vi "testGetConnStatusFromServersAandB.vi"(8 "error in":errorcluster) -> (0 "error out":errorcluster)   [LabVIEW 2018]
doc: "User can not get the connStatus boolean from two TCP/IP servers because runServer.vi can not run at same time."
uses:
  <vilib>/addons/_JKI Toolkits/Caraya/classes/Assert/Assert Equal Value_Variant.vi
  src/TcpServer/TcpServer.lvclass
  <vilib>/addons/_JKI Toolkits/Caraya/classes/Test/Test.lvclass
  <vilib>/addons/_JKI Toolkits/Caraya/classes/Assert/Assert.lvclass
panel:
  out "Run Server B error out":errorcluster
  out "Run Server A error out":errorcluster
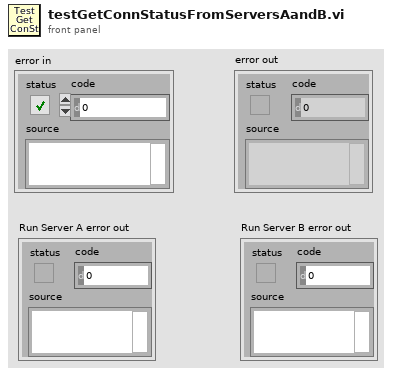
[diagram p1: front panel]
types:
  T1 = cluster{"CmdRead":refnum<user-event>, "EvtRead":refnum<user-event>, "GenRead":refnum<user-event>}
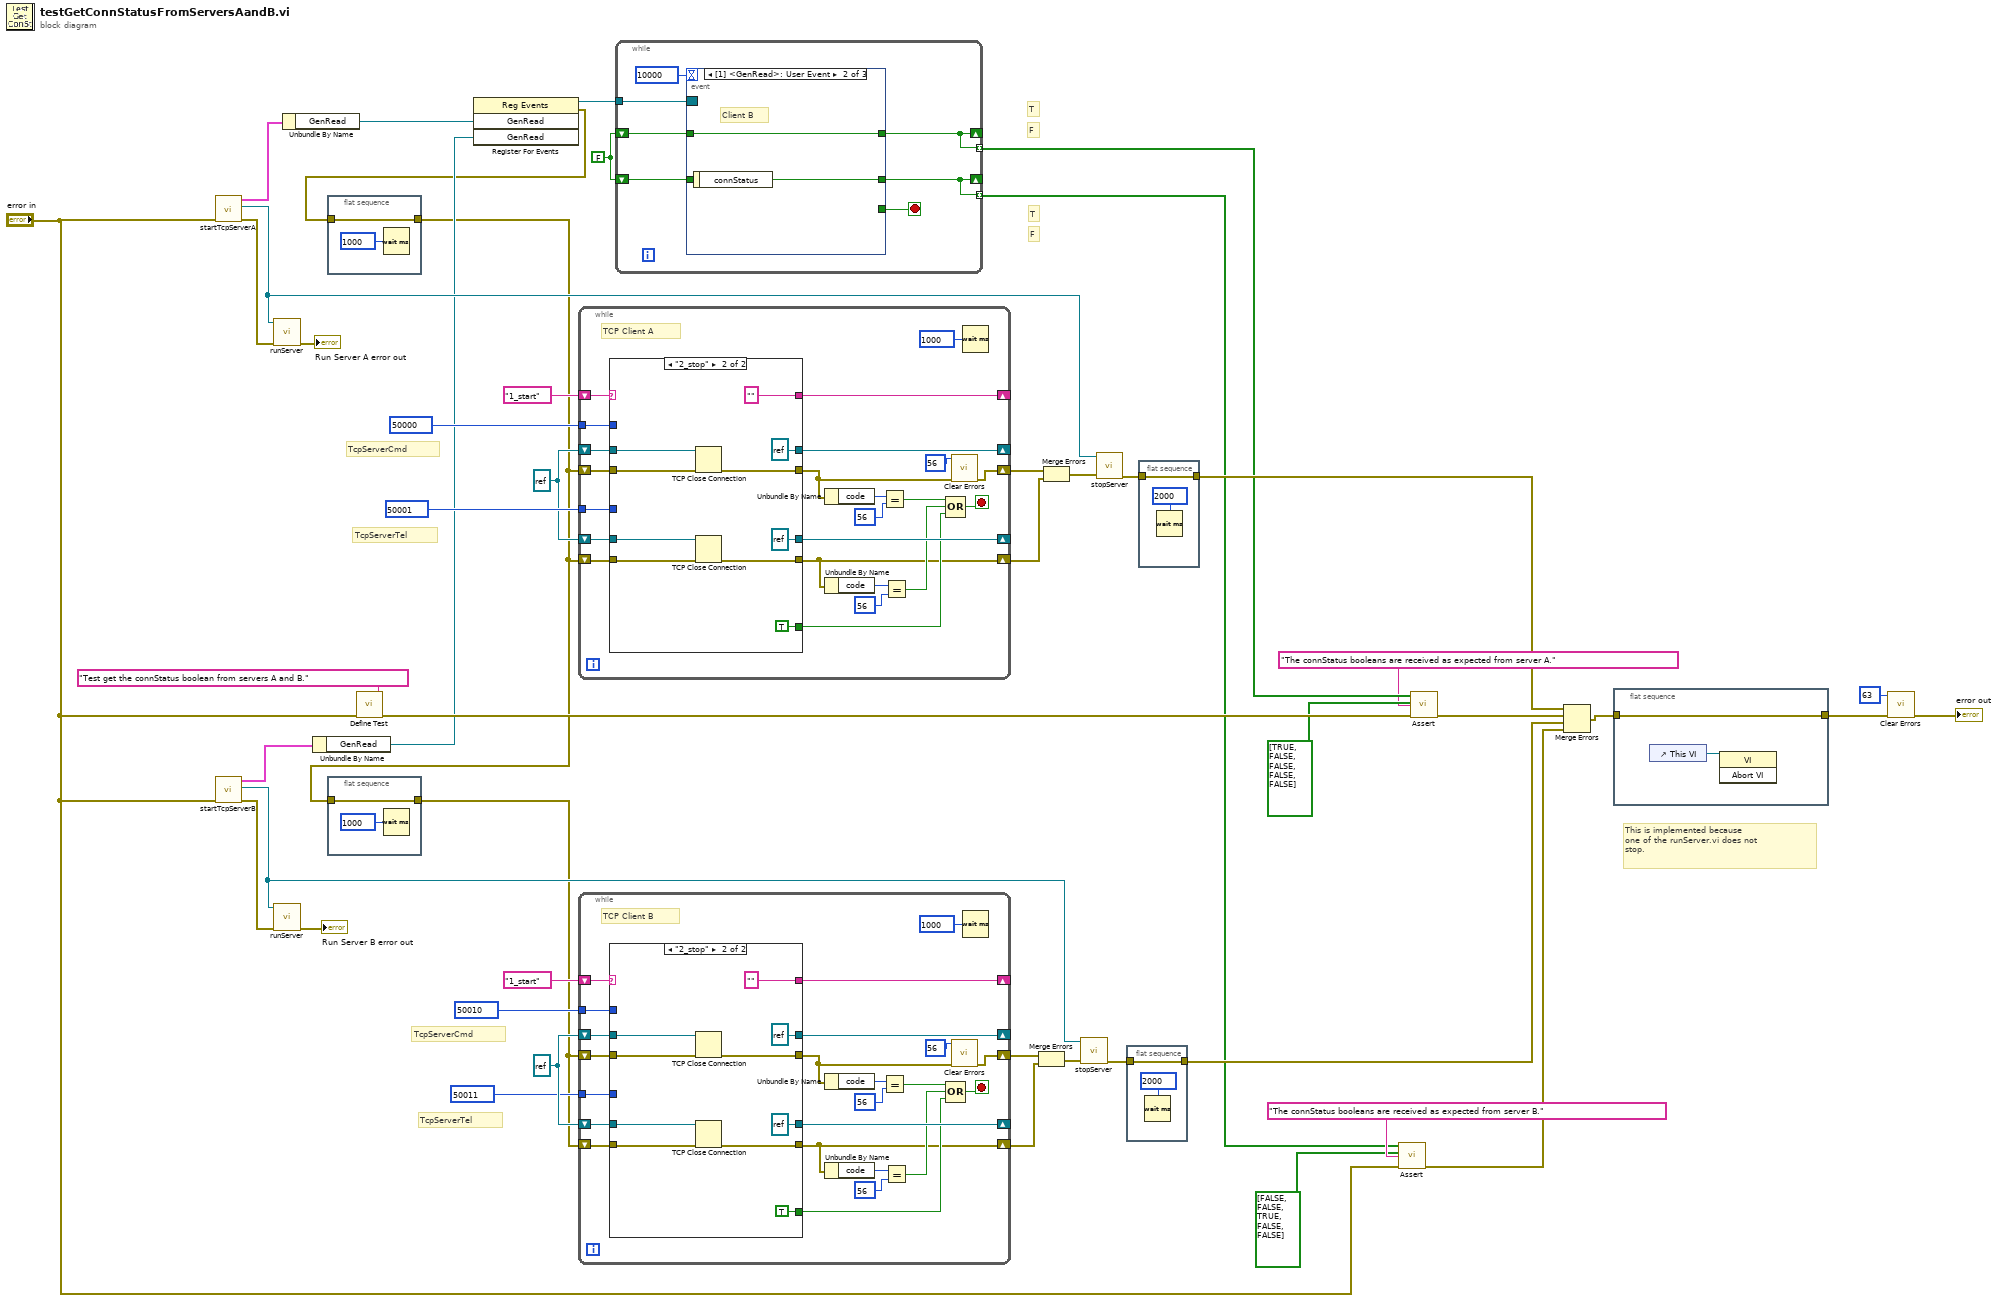
[diagram p0: block diagram]
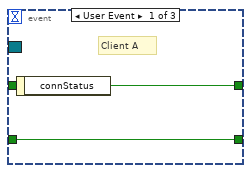
[diagram p2: hidden frame]
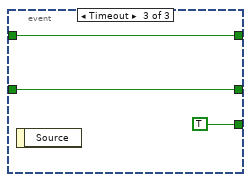
[diagram p3: hidden frame]
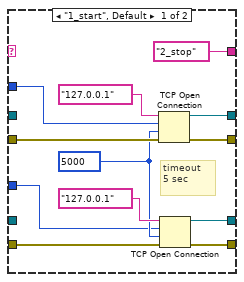
[diagram p4: hidden frame]
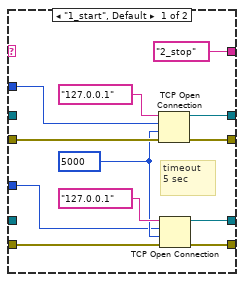
[diagram p5: hidden frame]
diagram:
  w18 = FALSE ("connStatus")
  w35 = refnum<k5> refnum ("connection ID")
  w37 = refnum<k5> refnum ("connection ID")
  # "F"
  # "F"
  # "T"
  # "T"
  # "This is implemented because\none of the runServer.vi does not\nstop."
  # "TcpServerTel"
  # "TcpServerCmd"
  # "TcpServerTel"
  # "TcpServerCmd"
  n1 = call "startTcpServerA.vi"("error in (no error)"="error in") -> ("error out"=w38:errorcluster, "TcpServer out"=w36:refnum<class "TcpServer.lvclass">, "UserEvents"=w24:T1)  [unwired: 8 in]
  n2 = call "startTcpServerB.vi"("error in (no error)"="error in") -> ("error out"=w26:errorcluster, "TcpServer out"=w28:refnum<class "TcpServer.lvclass">, "UserEvents"=w20:T1)  [unwired: 8 in]
  n3 = call "runServer.vi"("error in (no error)"=w38, "TcpServer in"=w36) -> ("error out (no error)"=→"Run Server A error out":errorcluster)  [unwired: 8 in, 1 out]
  n4 = call "runServer.vi"("error in (no error)"=w26, "TcpServer in"=w28) -> ("error out (no error)"=→"Run Server B error out":errorcluster)  [unwired: 8 in, 1 out]
  n5 = Unbundle By Name(w24) -> ("GenRead"=w23:refnum<user-event>)
  n6 = Unbundle By Name(w20) -> ("GenRead"=w19:refnum<user-event>)
  n7 = flat-sequence {
    tunnel: w7 -> [w49]
    tunnel: [w49] -> w6
    frame #0 {
      n8 = Wait (ms)(milliseconds to wait=u32 1000) -> ()  [unwired: 1 out]
    }
  }
  n9 = flat-sequence {
    tunnel: w6 -> [w51]
    tunnel: [w51] -> w27
    frame #0 {
      n10 = Wait (ms)(milliseconds to wait=u32 1000) -> ()  [unwired: 1 out]
    }
  }
  n11 = call <vilib>:"Define Test.vi"("error in (no error)"="error in", "Label (VI Title)"="Test get the connStatus boolean from servers A and B.") -> ("error out"=w40:errorcluster)  [unwired: 9 in]
  n12 = register-events(w23, w19) -> (reference out=w22:refnum<event-registration>, error out=w7:errorcluster)  [unwired: 2 in]
  n13 = while {
    shift-right: [w68] -> _
    shift-left: "1_start" ("address") -> [w75]
    shift-right: [w74] -> _
    shift-left: w37 -> [w72]
    shift-right: [w73] -> _
    shift-left: w37 -> [w71]
    shift-right: [w61] -> w44
    shift-left: w6 -> [w70]
    shift-right: [w56] -> w45
    shift-left: w6 -> [w69]
    tunnel: u16 50000 ("remote port or service name") -> [w54]
    tunnel: u16 50001 ("remote port or service name") -> [w53]
    stop <- w62 stop-if-true
    # "TCP Client A"
    n14 = case shown="\"2_stop\"" w75 {
      tunnel: [w85 refnum<k5> refnum ("connection ID")] -> w74
      tunnel: [w84 refnum<k5> refnum ("connection ID")] -> w73
      tunnel: w72 -> [_ w97]
      tunnel: w71 -> [_ w95]
      tunnel: [w83 w93] -> w58
      tunnel: [w82 w92] -> w56
      tunnel: w70 -> [w80 w96]
      tunnel: w69 -> [w79 w94]
      tunnel: ["2_stop" ("address") "" ("address")] -> w68
      tunnel: [_ TRUE] -> w59
      tunnel: w54 -> [w77 _]
      tunnel: w53 -> [w76 _]
      frame "1_start", Default {
        w78 = 5000 ("timeout ms (60000)")
        # "timeout\n5 sec"
        n15 = TCP Open Connection(address="127.0.0.1", remote port or service name=w77, timeout ms (60000)=w78, error in (no error)=w80) -> (connection ID=w85:refnum<k5>, error out=w83:errorcluster)  [unwired: 1 in]
        n16 = TCP Open Connection(address="127.0.0.1", remote port or service name=w76, timeout ms (60000)=w78, error in (no error)=w79) -> (connection ID=w84:refnum<k5>, error out=w82:errorcluster)  [unwired: 1 in]
      }
      frame "2_stop" {
        n17 = TCP Close Connection(connection ID=w97, error in (no error)=w96) -> (error out=w93:errorcluster)  [unwired: 1 in, 1 out]
        n18 = TCP Close Connection(connection ID=w95, error in (no error)=w94) -> (error out=w92:errorcluster)  [unwired: 1 in, 1 out]
      }
    }
    n19 = Unbundle By Name(w58) -> ("code"=w57:i32)
    n20 = Unbundle By Name(w56) -> ("code"=w55:i32)
    n21 = Equal?(x=w57, y=56) -> (x = y?=w64:bool)
    n22 = Equal?(x=w55, y=56) -> (x = y?=w63:bool)
    n23 = Compound Arithmetic op=OR(w64, w63, w59) -> (w62:bool)
    n24 = call <vilib>:"Clear Errors.vi"("error in (no error)"=w58, "specific error code to clear (0: all)"=56) -> ("error out"=w61:errorcluster)  [unwired: 4 in, 1 out]
    n25 = Wait (ms)(milliseconds to wait=u32 1000) -> ()  [unwired: 1 out]
  }
  n26 = while {
    shift-right: [w113] -> _
    shift-left: "1_start" ("address") -> [w120]
    shift-right: [w119] -> _
    shift-left: w35 -> [w117]
    shift-right: [w118] -> _
    shift-left: w35 -> [w116]
    shift-right: [w106] -> w32
    shift-left: w27 -> [w115]
    shift-right: [w101] -> w31
    shift-left: w27 -> [w114]
    tunnel: u16 50010 ("remote port or service name") -> [w99]
    tunnel: u16 50011 ("remote port or service name") -> [w98]
    stop <- w107 stop-if-true
    # "TCP Client B"
    n27 = case shown="\"2_stop\"" w120 {
      tunnel: [w130 refnum<k5> refnum ("connection ID")] -> w119
      tunnel: [w129 refnum<k5> refnum ("connection ID")] -> w118
      tunnel: w117 -> [_ w142]
      tunnel: w116 -> [_ w140]
      tunnel: [w128 w138] -> w103
      tunnel: [w127 w137] -> w101
      tunnel: w115 -> [w125 w141]
      tunnel: w114 -> [w124 w139]
      tunnel: ["2_stop" ("address") "" ("address")] -> w113
      tunnel: [_ TRUE] -> w104
      tunnel: w99 -> [w122 _]
      tunnel: w98 -> [w121 _]
      frame "1_start", Default {
        w123 = 5000 ("timeout ms (60000)")
        # "timeout\n5 sec"
        n28 = TCP Open Connection(address="127.0.0.1", remote port or service name=w122, timeout ms (60000)=w123, error in (no error)=w125) -> (connection ID=w130:refnum<k5>, error out=w128:errorcluster)  [unwired: 1 in]
        n29 = TCP Open Connection(address="127.0.0.1", remote port or service name=w121, timeout ms (60000)=w123, error in (no error)=w124) -> (connection ID=w129:refnum<k5>, error out=w127:errorcluster)  [unwired: 1 in]
      }
      frame "2_stop" {
        n30 = TCP Close Connection(connection ID=w142, error in (no error)=w141) -> (error out=w138:errorcluster)  [unwired: 1 in, 1 out]
        n31 = TCP Close Connection(connection ID=w140, error in (no error)=w139) -> (error out=w137:errorcluster)  [unwired: 1 in, 1 out]
      }
    }
    n32 = Unbundle By Name(w103) -> ("code"=w102:i32)
    n33 = Unbundle By Name(w101) -> ("code"=w100:i32)
    n34 = Equal?(x=w102, y=56) -> (x = y?=w109:bool)
    n35 = Equal?(x=w100, y=56) -> (x = y?=w108:bool)
    n36 = Compound Arithmetic op=OR(w109, w108, w104) -> (w107:bool)
    n37 = call <vilib>:"Clear Errors.vi"("error in (no error)"=w103, "specific error code to clear (0: all)"=56) -> ("error out"=w106:errorcluster)  [unwired: 4 in, 1 out]
    n38 = Wait (ms)(milliseconds to wait=u32 1000) -> ()  [unwired: 1 out]
  }
  n39 = while {
    tunnel: w22 -> [w149]
    tunnel: [w147] -> w14 mode=indexing
    tunnel: [w145] -> w3 mode=indexing
    shift-right: [w147] -> _
    shift-left: w18 -> [w146]
    shift-right: [w145] -> _
    shift-left: w18 -> [w144]
    stop <- w143 stop-if-true
    n40 = event shown="[1] <GenRead>: User Event" {
      selector: w149 -> [_ _ _]
      dyn-events: _ -> [_ _ _]
      timeout: 10000 -> [_ _ _]
      tunnel: [w151 w152 w156] -> w147
      tunnel: [w150 w153 w155] -> w145
      tunnel: w146 -> [_ w152 w156]
      tunnel: w144 -> [w150 _ w155]
      tunnel: [_ _ TRUE] -> w143
      event User Event {
        # "Client A"
        n41 = event-data() -> ("connStatus"=w151:bool)  [unwired: 1 in]
      }
      event User Event {
        # "Client B"
        n42 = event-data() -> ("connStatus"=w153:bool)  [unwired: 1 in]
      }
      event Timeout {
        n43 = event-data() -> ()  [unwired: 1 in, 1 out]
      }
    }
  }
  n44 = Merge Errors(w32, w31) -> (w33:errorcluster)
  n45 = Merge Errors(w44, w45) -> (w43:errorcluster)
  n46 = call "stopServer.vi"("error in (no error)"=w33, "tcpServer in"=w28) -> ("error out"=w25:errorcluster)  [unwired: 8 in, 1 out]
  n47 = call "stopServer.vi"("error in (no error)"=w43, "tcpServer in"=w36) -> ("error out"=w41:errorcluster)  [unwired: 8 in, 1 out]
  n48 = flat-sequence {
    tunnel: w25 -> [w157]
    tunnel: [w157] -> w15
    frame #0 {
      n49 = Wait (ms)(milliseconds to wait=u32 2000) -> ()  [unwired: 1 out]
    }
  }
  n50 = flat-sequence {
    tunnel: w41 -> [w159]
    tunnel: [w159] -> w16
    frame #0 {
      n51 = Wait (ms)(milliseconds to wait=u32 2000) -> ()  [unwired: 1 out]
    }
  }
  n52 = call-poly <vilib>:"Assert.vi"("Label"="The connStatus booleans are received as expected from server B.", "error in (no error)"="error in", "Y"=bool[] [FALSE, FALSE, TRUE, FALSE, FALSE], "X"=w3) -> ("error out"=w1:errorcluster)  [unwired: 7 in]
  n53 = call-poly <vilib>:"Assert.vi"("Label"="The connStatus booleans are received as expected from server A.", "error in (no error)"=w40, "Y"=bool[] [TRUE, FALSE, FALSE, FALSE, FALSE], "X"=w14) -> ("error out"=w39:errorcluster)  [unwired: 7 in]
  n54 = Merge Errors(w16, w39, w15, w1) -> (w17:errorcluster)
  n55 = flat-sequence {
    tunnel: w17 -> [w162]
    tunnel: [w162] -> w12
    frame #0 {
      n56 = control-ref of="This VI"() -> (w161:refnum<vi>)
      n57 = invoke class="VI" method="Abort VI"(reference=w161) -> ()  [unwired: 2 in, 3 out]
    }
  }
  n58 = call <vilib>:"Clear Errors.vi"("error in (no error)"=w12, "specific error code to clear (0: all)"=63) -> ("error out"=→"error out":errorcluster)  [unwired: 4 in, 1 out]
